vi "To Waveform.vi"(8 "error in (no error)":errorcluster, 11 "Double Array in":refnum<class "Double Array.lvclass">) -> (0 "error out":errorcluster, 1 "Success?":bool, 3 "Waveform Array":waveform(dbl)[](array[waveform]))   [LabVIEW 2020, in "Data.lvlib" / "Double Array.lvclass"]
doc: "Interpret 'Data' as a Waveform Array. If impossible 'Success?' is set to FALSE"
uses:
  Double Array.lvclass
  Double Array.lvclass/Double Array.ctl
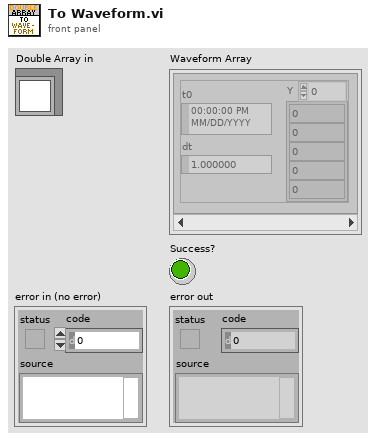
[diagram p1: front panel]
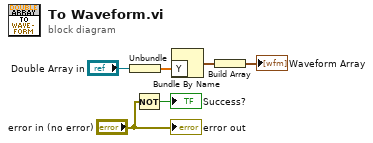
[diagram p0: block diagram]
diagram:
  n1 = Unbundle("Double Array in") -> (w4:dbl[])
  n2 = Not(x="error in (no error)") -> (.not. x?=→"Success?":bool)
  n3 = Bundle By Name("Y"=w4) -> (w6:waveform(dbl))  [unwired: 1 in]
  n4 = Build Array(w6) -> (→"Waveform Array":waveform(dbl)[])
  "error out" <- "error in (no error)"
